vi "Pre Launch Init.vi"(11 "Sample Error Reporter in":refnum<class "Sample Error Reporter.lvclass">) -> (0 "error out":errorcluster, 3 "Sample Error Reporter out":refnum<class "Sample Error Reporter.lvclass">)   [LabVIEW 2024, in "Sample Error Reporter.lvlib" / "Sample Error Reporter.lvclass"]
doc: "<p>(<strong>Filename</strong>: <span class=\"dnl\">Actor Framework.lvlib:Actor.lvclass:Pre Launch Init.vi</span>)</p>\n<p>Defines behavior that occurs after the <a href=\"nihelplauncher://docs/csh?context=lvcore_lvcomm_af_launch_nested_actor\">Launch Nested Actor</a> method is invoked but before the actor's Actor Core method begins running.</p>\n<p>By default, this method does nothing. A descendant class may override it to define behavior.</p>"
uses:
  Sample Error Reporter.lvclass
  Sample Error Reporter.lvclass/Sample Error Reporter.ctl
  src/Error Reporting Actor/Error Reporter/Error Reporter/Error Reporter.lvclass
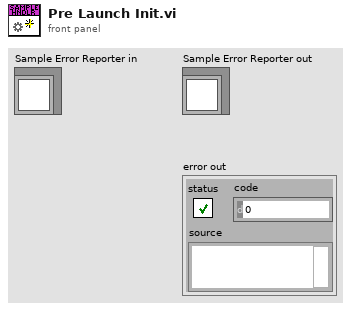
[diagram p1: front panel]
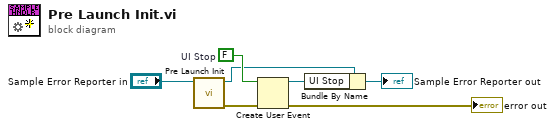
[diagram p0: block diagram]
diagram:
  w7 = FALSE  # UI Stop
  n1 = call-parent "Pre Launch Init.vi"("Actor in"="Sample Error Reporter in") -> ("error out"=w2:errorcluster, "Actor out"=w4:refnum<class "Sample Error Reporter.lvclass">)  [unwired: 9 in]
  n2 = Create User Event(user event datatype=w7, error in=w2) -> (user event=w6:refnum<user-event>, error out=→"error out":errorcluster)
  n3 = Bundle By Name(cluster=w4, "UI Stop"=w6) -> (→"Sample Error Reporter out":refnum<class "Sample Error Reporter.lvclass">)
